vi "Write Projects.vi"(8 "error in (no error)":errorcluster, 10 "Projects":string[](array[string]), 11 "DB in":refnum<class "DB.lvclass">) -> (0 "error out":errorcluster, 3 "DB out":refnum<class "DB.lvclass">)   [LabVIEW 2015, in "DB.lvclass"]
uses:
  DB.lvclass
  DB.lvclass/DB.ctl
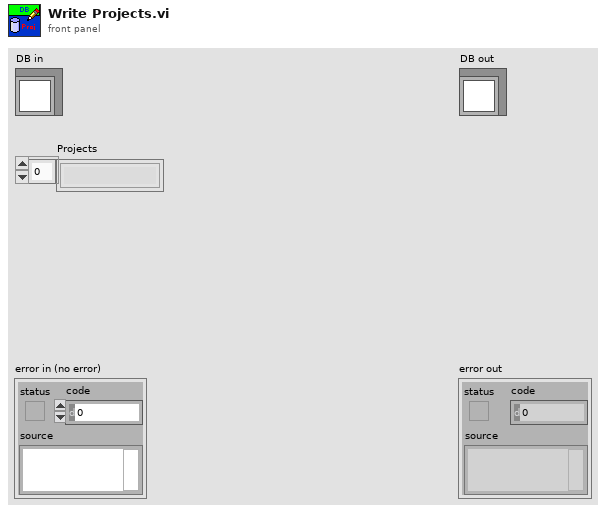
[diagram p1: front panel]
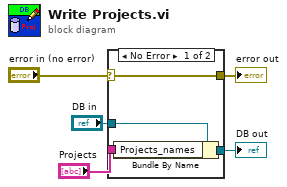
[diagram p0: block diagram]
diagram:
  n1 = case shown="No Error" "error in (no error)" {
    selector: "error in (no error)" -> [w9 w10]
    tunnel: [w9 w10] -> w4
    tunnel: [w7 w11] -> w2
    tunnel: "DB in" -> [w8 w11]
    tunnel: "Projects" -> [w6 _]
    frame No Error {
      n2 = Bundle By Name(cluster=w8, "Projects_names"=w6) -> (w7:refnum<class "DB.lvclass">)
    }
    frame Error {
    }
  }
  "error out" <- w4
  "DB out" <- w2
